vi "Data Correction.vi"(8 "error in (no error)":errorcluster, 10 "Input onfiguration":T1 {"Offset" scale=0.0..0.1; "Scale" scale=0.0..0.03; "Model parameters"."Resolution" format="%#_6peV"; "Model parameters"."Integration range" format="%#_6peV"; "Model parameters"."T" format="%#_6pK"; "Model parameters"."Delta" step=0.001 format="%#_6peV"; "Model parameters"."Gama" step=0.001 format="%#_6peV"; "Resistance in series" scale=0.0..80.0}, 11 "dIdV State in":refnum<class "dIdV State.lvclass">) -> (0 "error out":errorcluster, 3 "dIdV State out":refnum<class "dIdV State.lvclass">)   [LabVIEW 2021, in "dIdV State.lvclass"]
uses:
  dIdV State.lvclass
  Controls/PCS Config.ctl
  Parameters.ctl
  dIdV State.lvclass/dIdV State.ctl
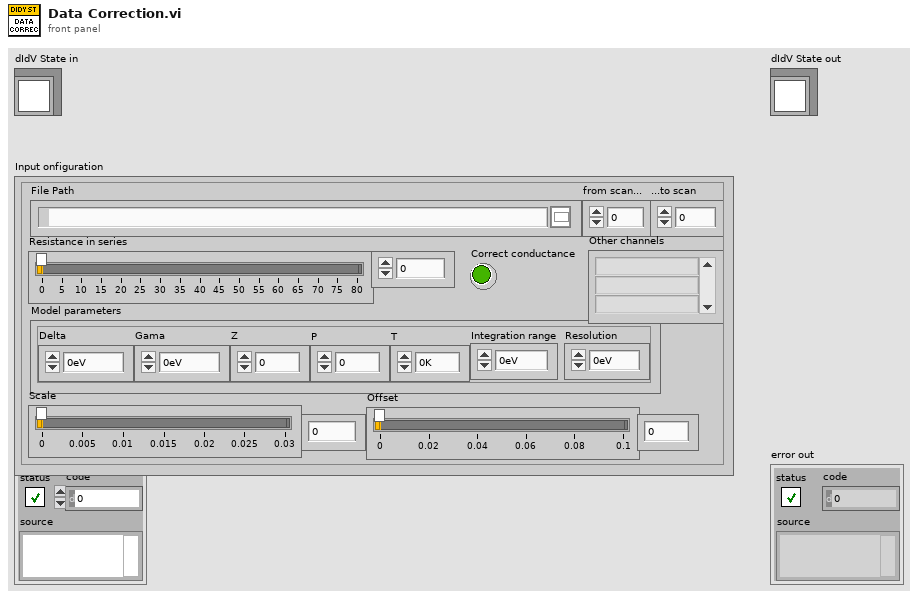
[diagram p1: front panel]
types:
  T1 = typedef "PCS Config.ctl" = cluster{"File Path":path, "from scan...":i32, "...to scan":i32, "Resistance in series":dbl, "Correct conductance ":bool, "Model parameters":T2, "Scale":dbl, "Offset":dbl, "Other channels":string[]}
  T2 = typedef "Parameters.ctl" = cluster{"Delta":dbl, "Gama":dbl, "Z":dbl, "P":dbl, "T":dbl, "Integration range":dbl, "Resolution":dbl}
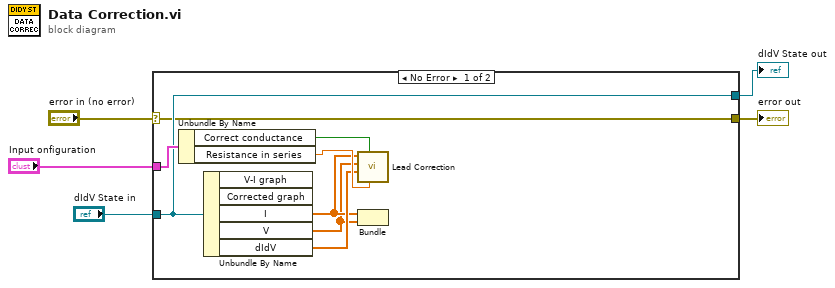
[diagram p0: block diagram]
diagram:
  n1 = case shown="No Error" "error in (no error)" {
    selector: "error in (no error)" -> [w8 w15]
    tunnel: [w8 w15] -> w4
    tunnel: [w11 w14] -> w2
    tunnel: "dIdV State in" -> [w11 w14]
    tunnel: "Input onfiguration" -> [w13 _]
    frame No Error {
      n2 = Unbundle By Name(w13) -> ("Correct conductance"=w9:bool, "Resistance in series"=w12:dbl)
      n3 = Unbundle By Name(w11) -> ("I"=w7:dbl[], "V"=w6:dbl[], "dIdV"=w10:dbl[])  [unwired: 2 out]
      n4 = call "Lead Correction.vi"("Resistance in series"=w12, "Correct conductance"=w9, "dIdV"=w10, "V"=w6, "I"=w7) -> ()  [unwired: 3 in, 4 out]
      n5 = Bundle("I"=w7, "V"=w6) -> ()  [unwired: 1 in, 1 out]
    }
    frame Error {
    }
  }
  "error out" <- w4
  "dIdV State out" <- w2
